vi "LIA_DAQ_Main(trigger).vi"() -> ()   [LabVIEW 2016, in "ZI LIA.lvlib"]
doc: "Control a Zurich instrument device via the LabOne Labview API. \nRequirements: Zurich Instruments MFLI, HF2 or UHFLI \nThis example shows how to start a DAQ trigger module and retrieve the Data.\n\n© Zurich Instruments AG, www.zhinst.com"
uses:
  ZI LIA.lvlib
  Ctl_SetParameter(Value).ctl
  <instrlib>/Zurich Instruments LabOne/Public/Modules/ziModSetValueBinaryArray.vi
  <instrlib>/Zurich Instruments LabOne/Zurich Instruments LabOne.lvlib
  General.lvlib
panel:
  out "error out":errorcluster
  out "Waveform Graph":dbl[][](graph)
  out "Grid DEMOD R":dbl[][](array[numeric])
  in  "Address":string="DEV2090"
  out "Selected Device":string
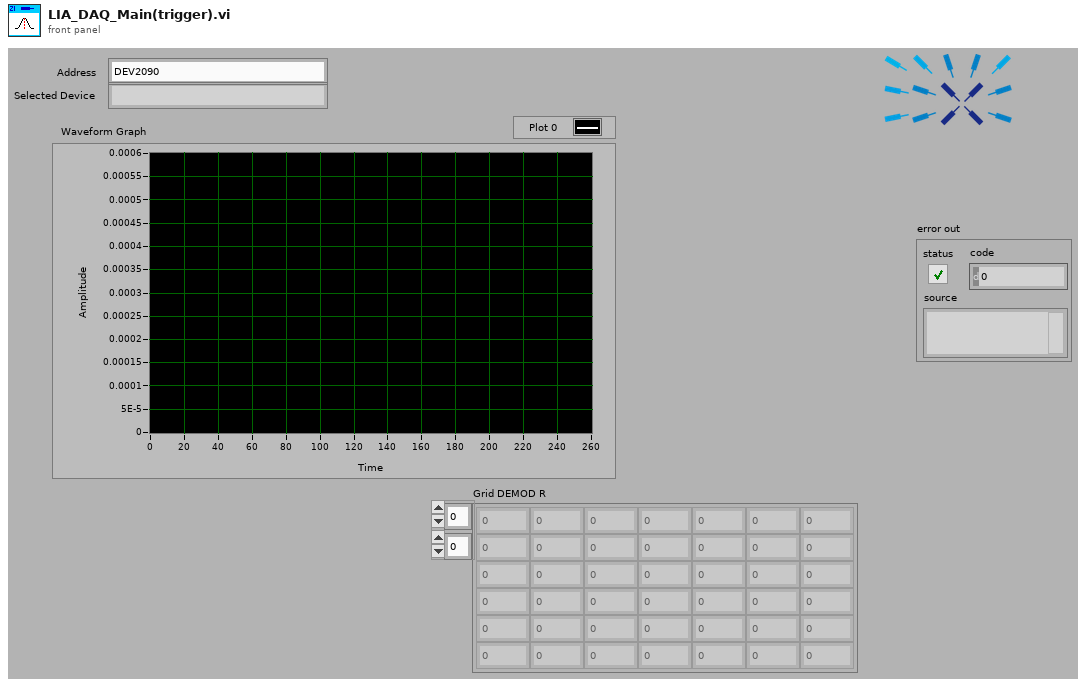
[diagram p1: front panel]
types:
  T1 = typedef "General.lvlib/Ctl_SetParameter(Value).ctl" = cluster{"Path":string, "Value":dbl, "comment":string}
  T2 = typedef "Zurich Instruments LabOne.lvlib/ziTypeModHandle.ctl" = cluster{"handleValid":bool, "Conn":u64, "ModHandle":u64, "moduleID":string, "Path Prefix":string}
  T3 = typedef "Zurich Instruments LabOne.lvlib/ziTypeHandle.ctl" = cluster{"handleValid":bool, "Conn":u64, "Path Prefix":string, "Handle":u64, "Connected":bool, "Clockbase(s)":dbl}
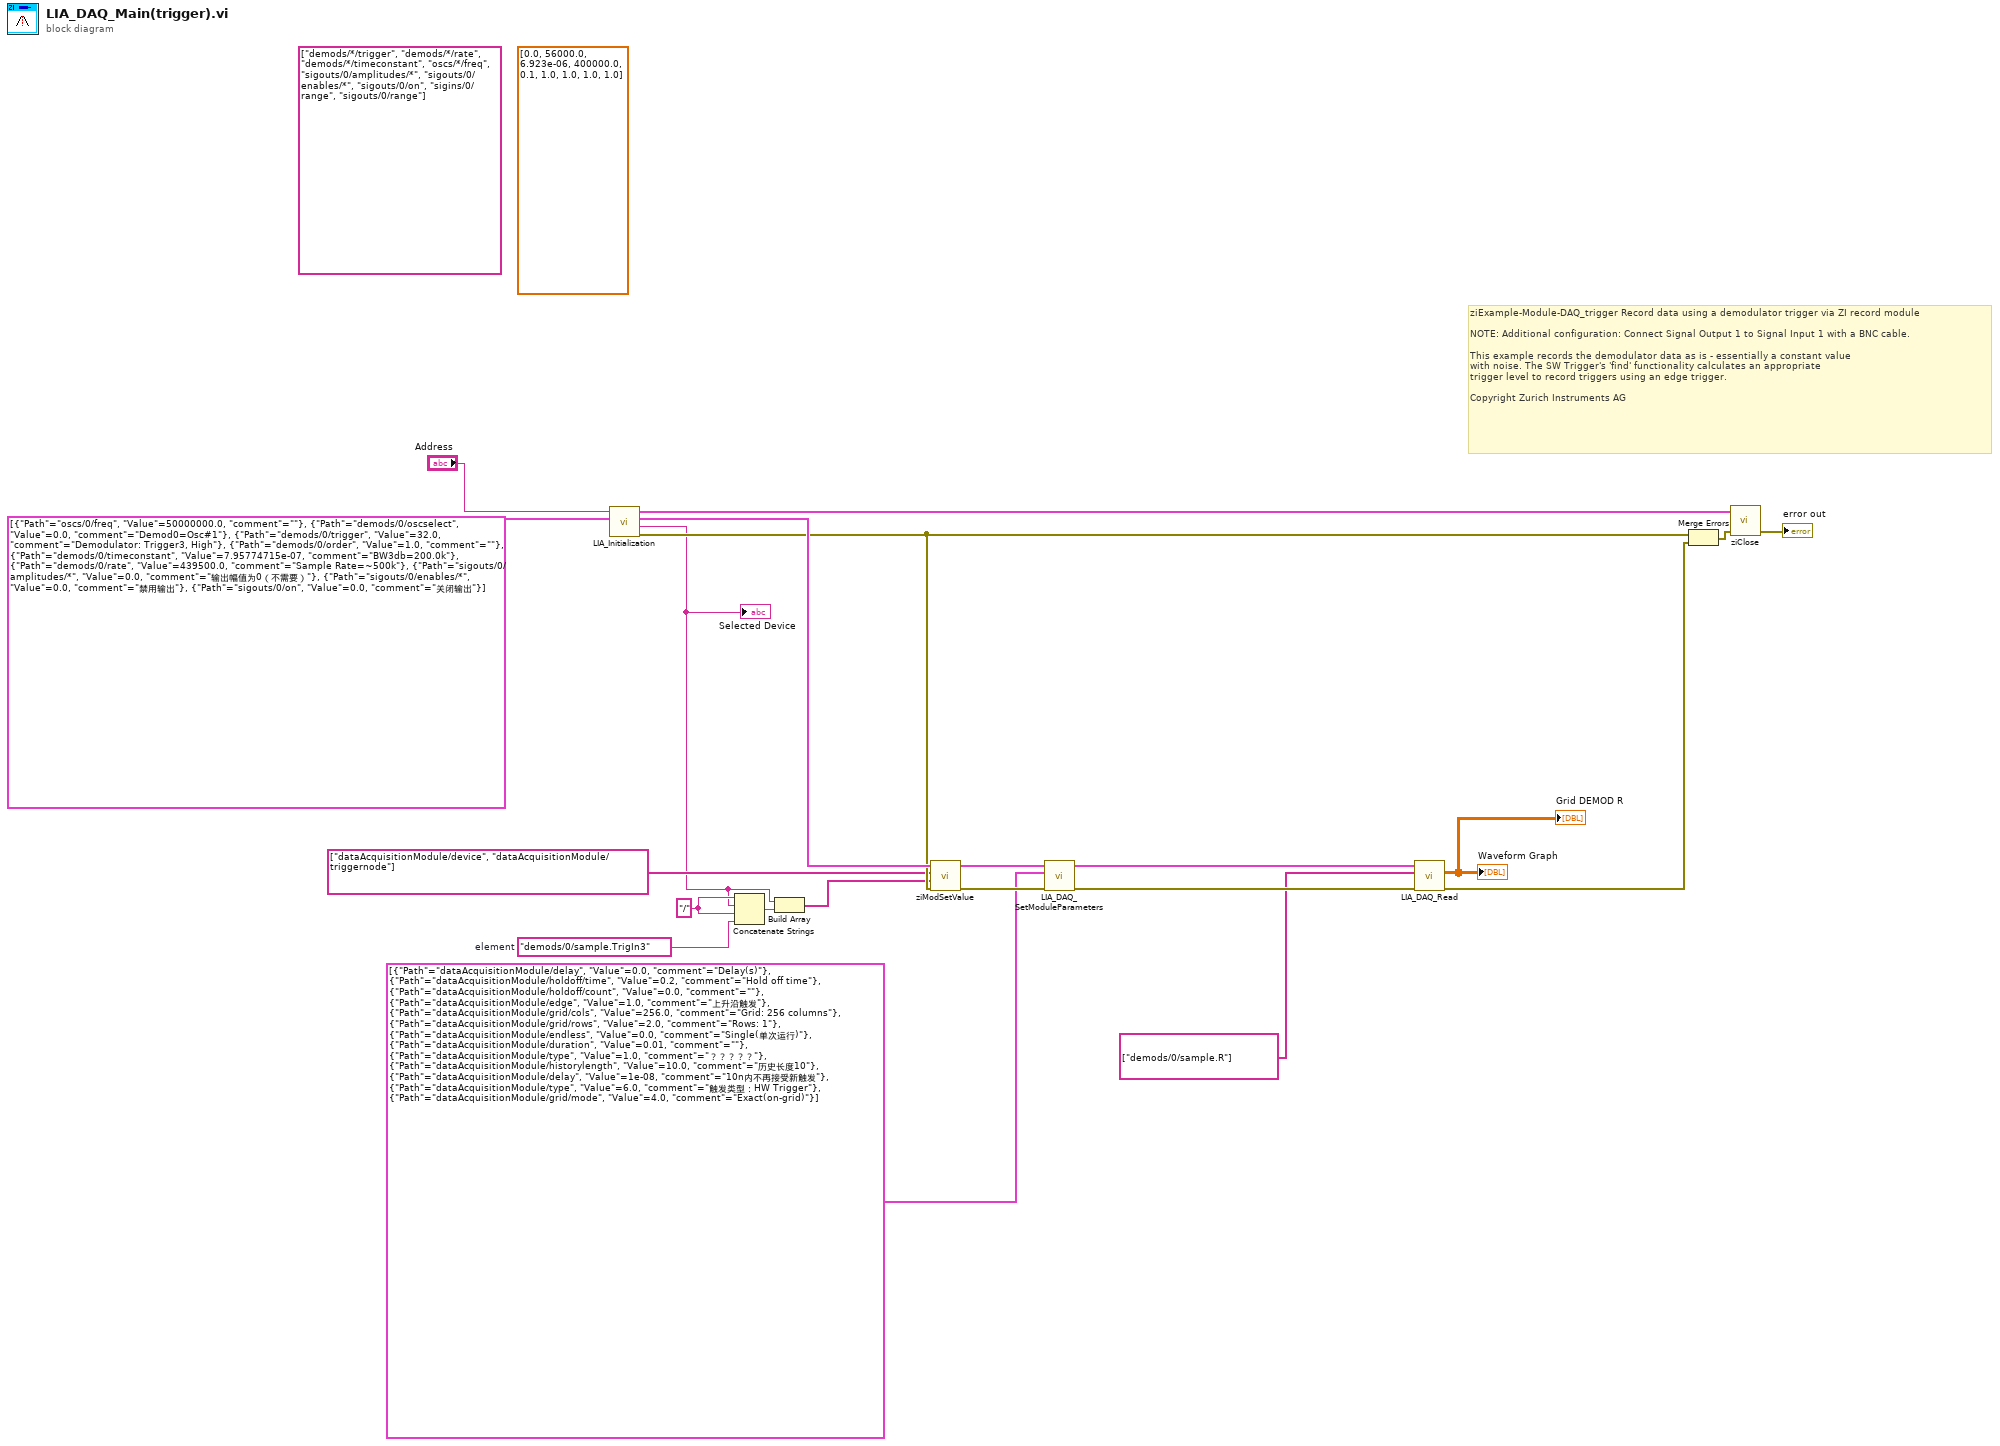
[diagram p0: block diagram]
diagram:
  w9 = "/"
  w10 = "demods/0/sample.TrigIn3"  # element
  (unwired) dbl[] [0.0, 56000.0, 6.923e-06, 400000.0, 0.1, 1.0, 1.0, 1.0, 1.0]
  (unwired) string[] ["demods/*/trigger", "demods/*/rate", "demods/*/timeconstant", "oscs/*/freq", "sigouts/0/amplitudes/*", "sigouts/0/enables/*", "sigouts/0/on", "sigins/0/range", "sigouts/0/range"]
  # "ziExample-Module-DAQ_trigger Record data using a demodulator trigger via ZI record module\n \nNOTE: Additional configuration: Connect Signal Output 1 to Signal Input 1 with a BNC cable.\n\nThis example records the demodulator data as is - essentially a constant value\nwith noise. The SW Trigger's 'find' functionality calculates an appropriate\ntrigger level to record triggers using an edge trigger.\n\nCopyright Zurich Instruments AG"
  n1 = call "LIA_Initialization.vi"("Lock-in Parameters"=T1[] [{"Path"="oscs/0/freq", "Value"=50000000.0, "comment"=""}, {"Path"="demods/0/oscselect", "Value"=0.0, "comment"="Demod0=Osc#1"}, {"Path"="demods/0/trigger", "Value"=32.0, "comment"="Demodulator: Trigger3, High"}, {"Path"="demods/0/order", "Value"=1.0, "comment"=""}, {"Path"="demods/0/timeconstant", "Value"=7.95774715e-07, "comment"="BW3db=200.0k"}, {"Path"="demods/0/rate", "Value"=439500.0, "comment"="Sample Rate=~500k"}, {"Path"="sigouts/0/amplitudes/*", "Value"=0.0, "comment"="输出幅值为0（不需要）"}, {"Path"="sigouts/0/enables/*", "Value"=0.0, "comment"="禁用输出"}, {"Path"="sigouts/0/on", "Value"=0.0, "comment"="关闭输出"}], "Address"="Address") -> ("error out"=w18:errorcluster, "Selected Device"=w8:string, "DAQ ModHandle Out"=w21:T2, "Handle Out"=w17:T3)  [unwired: 6 in]
  "Selected Device" <- w8
  n2 = Concatenate Strings(w9, w8, w9, w10) -> (w7:string)
  n3 = Build Array(w8, w7) -> (w16:string[])
  n4 = call-poly <instrlib>:"ziModSetValue.vi"("Error In"=w18, "Values"=w16, "Paths"=string[] ["dataAcquisitionModule/device", "dataAcquisitionModule/triggernode"], "ModHandle In"=w21) -> ("Error Out"=w13:errorcluster, "ModHandle Out"=w14:T2)  [unwired: 6 in]
  n5 = call "LIA_DAQ_SetModuleParameters.vi"("error in (no error)"=w13, "LIA DAQ Module Parameters"=T1[] [{"Path"="dataAcquisitionModule/delay", "Value"=0.0, "comment"="Delay(s)"}, {"Path"="dataAcquisitionModule/holdoff/time", "Value"=0.2, "comment"="Hold off time"}, {"Path"="dataAcquisitionModule/holdoff/count", "Value"=0.0, "comment"=""}, {"Path"="dataAcquisitionModule/edge", "Value"=1.0, "comment"="上升沿触发"}, {"Path"="dataAcquisitionModule/grid/cols", "Value"=256.0, "comment"="Grid: 256 columns"}, {"Path"="dataAcquisitionModule/grid/rows", "Value"=2.0, "comment"="Rows: 1"}, {"Path"="dataAcquisitionModule/endless", "Value"=0.0, "comment"="Single(单次运行)"}, {"Path"="dataAcquisitionModule/duration", "Value"=0.01, "comment"=""}, {"Path"="dataAcquisitionModule/type", "Value"=1.0, "comment"="？？？？？"}, {"Path"="dataAcquisitionModule/historylength", "Value"=10.0, "comment"="历史长度10"}, {"Path"="dataAcquisitionModule/delay", "Value"=1e-08, "comment"="10n内不再接受新触发"}, {"Path"="dataAcquisitionModule/type", "Value"=6.0, "comment"="触发类型：HW Trigger"}, {"Path"="dataAcquisitionModule/grid/mode", "Value"=4.0, "comment"="Exact(on-grid)"}], "DAQ ModHandle In"=w14) -> ("error out"=w11:errorcluster, "DAQ ModHandle Out"=w12:T2)  [unwired: 7 in]
  n6 = call "LIA_DAQ_Read.vi"("error in (no error)"=w11, "Subscribe Path Array"=string[] ["demods/0/sample.R"], "DAQ ModHandle In"=w12) -> ("error out"=w20:errorcluster, "Grid DEMOD R"=→"Waveform Graph" →"Grid DEMOD R":dbl[][])  [unwired: 6 in, 1 out]
  n7 = Merge Errors(w18, w20) -> (w19:errorcluster)
  n8 = call <instrlib>:"ziClose.vi"("Error In"=w19, "Handle In"=w17) -> ("Error Out"=→"error out":errorcluster)  [unwired: 2 in, 1 out]
